vi "Create From Matrix.vi"(8 "error in":errorcluster, 10 "Rotation Matrix":T1=[[1.0, 0.0, 0.0], [0.0, 1.0, 0.0], [0.0, 0.0, 1.0]]) -> (0 "error out":errorcluster, 3 "Orient3d out":refnum<class "Orient3d Class.lvclass">)   [LabVIEW 2011, in "Orient3d Class.lvclass"]
uses:
  Orient3d Class.lvclass
  <vilib>/Analysis/Matrix/Datatypes/RealMatrix.ctl
  Orient3d Class.lvclass/Orient3d Class.ctl
  <vilib>/imath/engines/lvmath2/RunTimeEngine/ErrorHandling/NIMS_Finalize Error.vi
  <vilib>/Analysis/Matrix/Numeric/Conversions/Matrix To Array - RM.vi
  <vilib>/imath/engines/lvmath2/RunTimeEngine/VariableToken/Read/NIMS_Get Elements - SorM(_,_) - Check - Check.vi
  <instcachedir>/0/NIMS_Get Elements - SorM(_,_) - Check - Check_DA1E252EAB634D989357E7C72E8137F5.lvgen/NIMS_Get Elements - SorM(_,_) - Check - Check_DA1E252EAB634D989357E7C72E8137F5_001.vi
  <vilib>/imath/engines/lvmath2/RunTimeEngine/ErrorHandling/NIMS_Create Error From Enums.vi
  <vilib>/imath/engines/lvmath2/RunTimeEngine/NodeEndStatement/NIMS_NodeEndStatement_Output.vi
  <instcachedir>/0/NIMS_NodeEndStatement_Output_53EC0D466D134D7ABD903AC30B43404B.lvgen/NIMS_NodeEndStatement_Output_53EC0D466D134D7ABD903AC30B43404B_002.vi
  <vilib>/Analysis/Matrix/NI_Matrix.lvlib
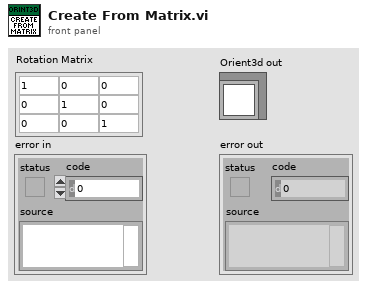
[diagram p1: front panel]
types:
  T1 = typedef "NI_Matrix.lvlib/RealMatrix.ctl" = dbl[][]
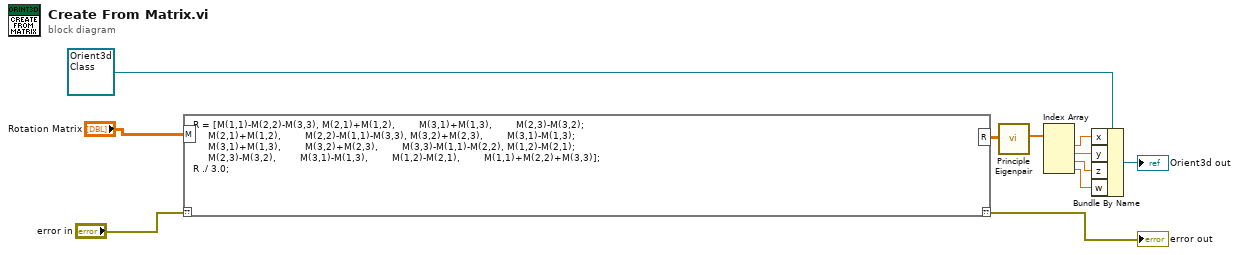
[diagram p0: block diagram]
diagram:
  n1 = mathscript code="R = [M(1,1)-M(2,2)-M(3,3), M(2,1)+M(1,2),        M(3,1)+M(1,3),        M(2,3)-M(3,2);\n     M(2,1)+M(1,2),        M(2,2)-M(1,1)-M(3,3), M(3,2)+M(2,3),        M(3,1)-M(1,3);\n     M(3,1)+M(1,3),        M(3,2)+M(2,3),        M(3,3)-M(1,1)-M(2,2), M(1,2)-M(2,1);\n     M(2,3)-M(3,2),        M(3,1)-M(1,3),        M(1,2)-M(2,1),        M(1,1)+M(2,2)+M(3,3)];\nR ./ 3.0;"("??"="error in", "M"="Rotation Matrix") -> ("??"=→"error out":errorcluster, "R"=w6:dbl[][])
  n2 = call "Principle Eigenpair.vi"("Matrix"=w6) -> ("Principal Eigenvector"=w5:dbl[])  [unwired: 9 in, 1 out]
  n3 = Index Array(array=w5) -> (element #1=w4:dbl, element #2=w3:dbl, element #3=w2:dbl, element #4=w1:dbl)  [unwired: 4 in]
  n4 = Bundle By Name(cluster=refnum<class "Orient3d Class.lvclass"> refnum ("Orient3d Class in"), "x"=w4, "y"=w3, "z"=w2, "w"=w1) -> (→"Orient3d out":refnum<class "Orient3d Class.lvclass">)
